vi "FrictionCompensation.vi"(8 "REV Compensation":u16, 9 "FWD Compensation":u16, 11 "Input":u16) -> (3 "Output":u16)   [LabVIEW 2013, in "ProcessorHelperFunctions.lvlib"]
uses:
  ProcessorHelperFunctions.lvlib
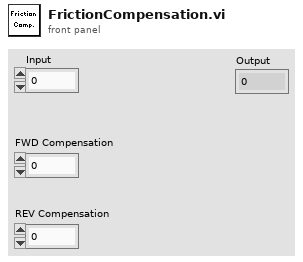
[diagram p1: front panel]
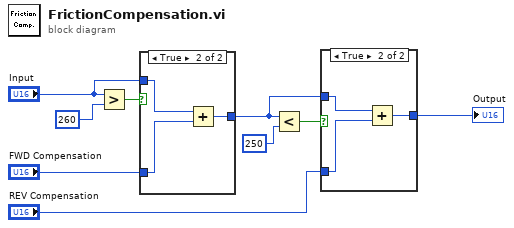
[diagram p0: block diagram]
diagram:
  n1 = Greater?(x="Input", y=u16 260) -> (0:w8:bool)
  n2 = case shown="True" w8 {
    tunnel: "Input" -> [w10 w13]
    tunnel: "FWD Compensation" -> [_ w12]
    tunnel: [w10 w11] -> w2
    frame False {
    }
    frame True {
      n3 = Add(x=w13, y=w12) -> (x+y=w11:u16)
    }
  }
  n4 = Less?(x=w2, y=u16 250) -> (x < y?=w4:bool)
  n5 = case shown="True" w4 {
    tunnel: "REV Compensation" -> [_ w16]
    tunnel: w2 -> [w14 w17]
    tunnel: [w14 w15] -> w1
    frame False {
    }
    frame True {
      n6 = Add(x=w17, y=w16) -> (x+y=w15:u16)
    }
  }
  "Output" <- w1
